vi "ukol1.vi"() -> ()   [LabVIEW 2023]
panel:
  out "text":string
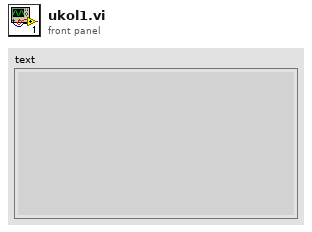
[diagram p1: front panel]
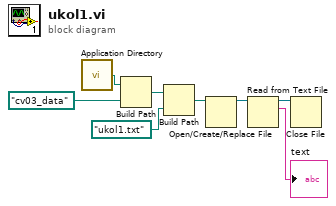
[diagram p0: block diagram]
diagram:
  n1 = call <vilib>:"Application Directory.vi"() -> ("Application Directory"=w8:path)
  n2 = Build Path(base path=w8, name or relative path=path "cv03_data") -> (appended path=w7:path)
  n3 = Build Path(base path=w7, name or relative path=path "ukol1.txt") -> (appended path=w3:path)
  n4 = Open/Create/Replace File(file path (use dialog)=w3) -> (refnum out=w2:refnum<file>)  [unwired: 5 in, 2 out]
  n5 = Read from Text File(file (use dialog)=w2) -> (refnum out=w1:refnum<file>, text=→"text":string)  [unwired: 3 in, 2 out]
  n6 = Close File(refnum=w1) -> ()  [unwired: 1 in, 2 out]
